vi "02_array.vi"(8 "errorIn":errorcluster, 11 "ArrayIn":i32[](array[numeric])=[0, 0, 0, 0]) -> (0 "errorOut":errorcluster, 3 "ArrayOut":i32[](array[numeric]))   [LabVIEW 2011]
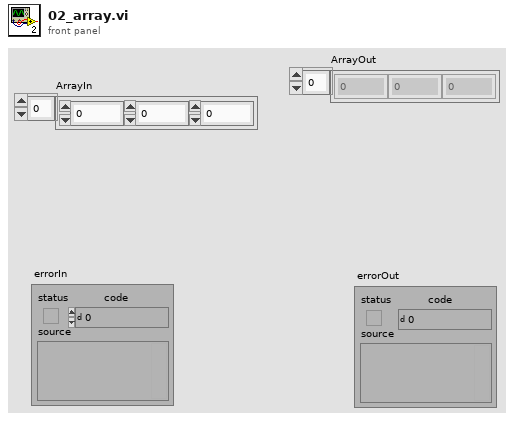
[diagram p1: front panel]
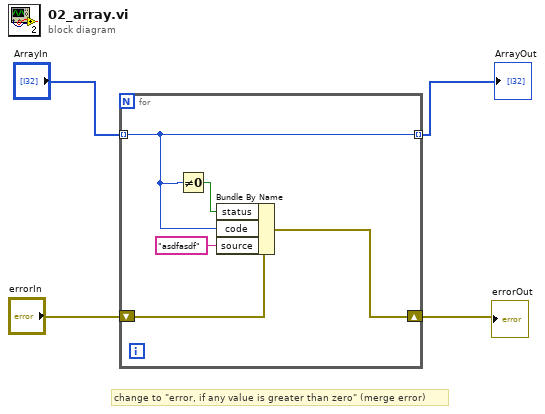
[diagram p0: block diagram]
diagram:
  # "change to \"error, if any value is greater than zero\" (merge error)"
  n1 = for {
    tunnel: "ArrayIn" -> [w7] mode=indexing
    shift-right: [w5] -> w3
    shift-left: "errorIn" -> [w6]
    tunnel: [w7] -> w1 mode=indexing
    n2 = Not Equal To 0?(x=w7) -> (x != 0?=w8:bool)
    n3 = Bundle By Name(cluster=w6, "status"=w8, "code"=w7, "source"="asdfasdf") -> (w5:errorcluster)
  }
  "ArrayOut" <- w1
  "errorOut" <- w3
